vi "Table, Get Column Value, String.vi"(0 "error in":errorcluster, 3 "Tbl Refnum":refnum<vi>, 4 "column (0)":i32) -> (7 "error out":errorcluster, 9 "Value":string[](array[string]), 10 "Tbl Refnum out":refnum<vi>)   [LabVIEW 2010]
doc: "This function gets a single column in string format from a table."
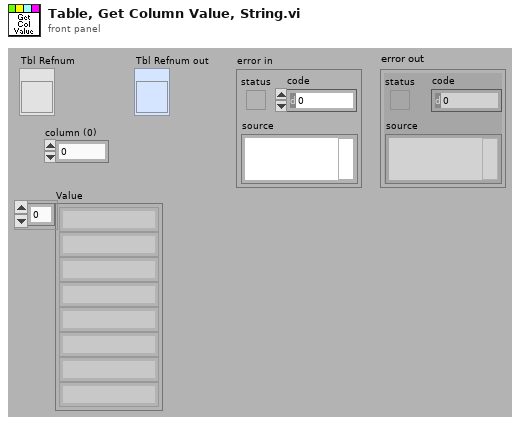
[diagram p1: front panel]
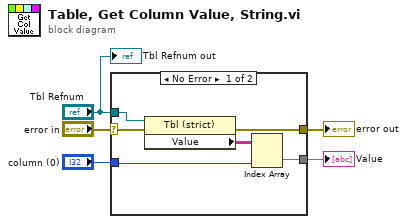
[diagram p0: block diagram]
diagram:
  n1 = case shown="No Error" "error in" {
    selector: "error in" -> [w10 w12]
    tunnel: "Tbl Refnum" -> [w11 _]
    tunnel: [w7 w12] -> w5
    tunnel: "column (0)" -> [w8 _]
    tunnel: [w6 _] -> w1
    frame No Error {
      n2 = property class="Tbl (strict)"(reference=w11, error in=w10) -> (error out=w7:errorcluster, "Value"=w9:string[][])  [unwired: 1 out]
      n3 = Index Array(array=w9, index (col)=w8) -> (element=w6:string[])  [unwired: 1 in]
    }
    frame Error {
    }
  }
  "error out" <- w5
  "Value" <- w1
  "Tbl Refnum out" <- "Tbl Refnum"
